vi "Log_Pictures.vi"   [LabVIEW 2017]
uses:
  Anemometry Sub Vis/Controls/Post_Process.ctl
  Anemometry Sub Vis/Globals/Preference_global.vi
  Anemometry Sub Vis/Globals/Extra_Commands_Global.vi
  Anemometry Sub Vis/Globals/Meas_global.vi
  Anemometry Sub Vis/Globals/Trav_pos_global.vi
types:
  T1 = typedef "Post_Process.ctl" = enum16{"Take New Data", "Post Process Raw Data File"}
  T2 = typedef "Camera resolution.ctl" = u8
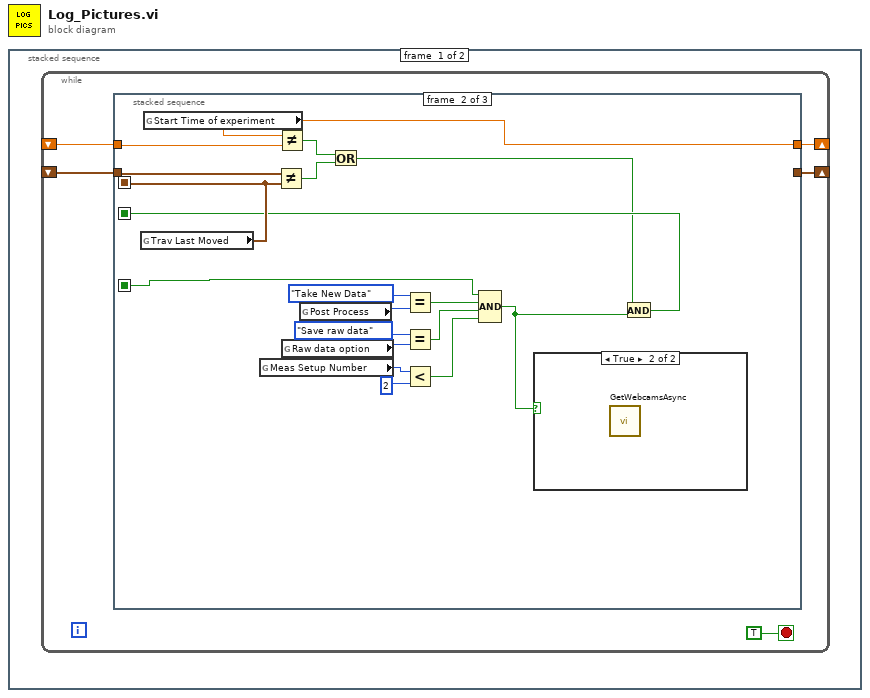
[diagram p0: block diagram]
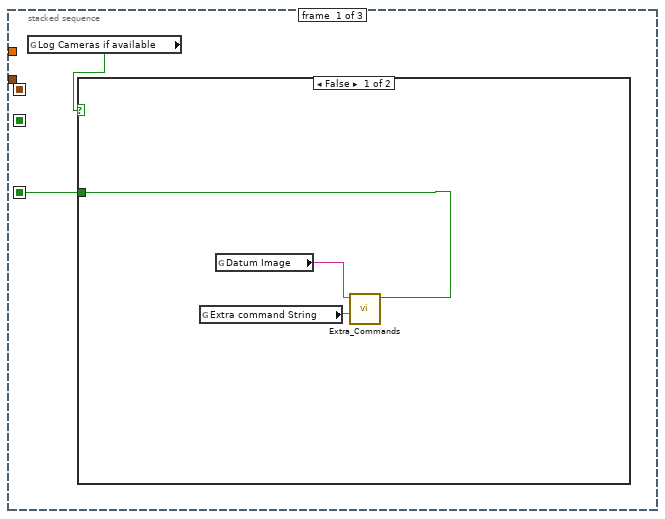
[diagram p2: hidden frame]
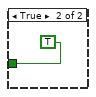
[diagram p3: hidden frame]
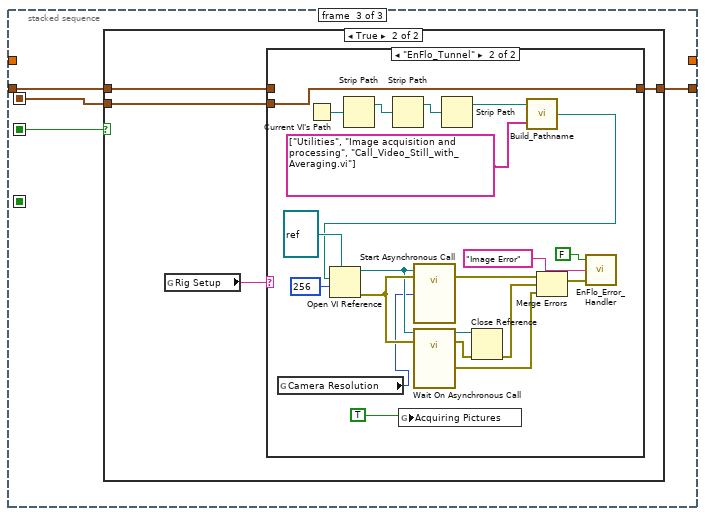
[diagram p5: hidden frame]
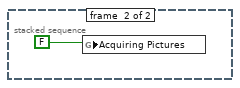
[diagram p8: hidden frame]
diagram:
  n1 = stacked-sequence {
    frame #0 {
      n2 = while {
        shift-right: [w5] -> _
        shift-left: _ -> [w4]
        shift-right: [w2] -> _
        shift-left: _ -> [w3]
        stop <- TRUE stop-if-true
        n3 = stacked-sequence {
          seq-local: [_ w15 _] -> [_ _ w34]
          seq-local: [_ w18 _] -> [_ _ w31]
          seq-local: [w6 _ _] -> [_ w12 _]
          tunnel: [_ _ w33] -> w5
          tunnel: w4 -> [_ w22 w32]
          tunnel: w3 -> [_ w21 _]
          tunnel: [_ w17 _] -> w2
          frame #0 {
            n4 = global read "Preference_global.vi" "Log Cameras if available"() -> (w7:bool)
            n5 = case shown="False" w7 {
              tunnel: [w8 TRUE] -> w6
              frame False {
                n6 = global read "Meas_global.vi" "Extra command String"() -> (w10:string)
                n7 = global read "Extra_Commands_Global.vi" "Datum Image"() -> (w9:string)
                n8 = call "Extra_Commands.vi"("String to Search"=w10, "Command"=w9) -> ("Command Found"=w8:bool)  [unwired: 2 in, 3 out]
              }
              frame True {
              }
            }
          }
          frame #1 {
            n9 = global read "Trav_pos_global.vi" "Trav Last Moved"() -> (w18:timestamp)
            n10 = global read "Meas_global.vi" "Start Time of experiment"() -> (w17:dbl)
            n11 = global read "Trav_pos_global.vi" "Meas Setup Number"() -> (w24:i32)
            n12 = Not Equal?(x=w22, y=w18) -> (x != y?=w19:bool)
            n13 = Not Equal?(x=w17, y=w21) -> (x != y?=w20:bool)
            n14 = global read "Meas_global.vi" "Raw data option"() -> (w27:enum16{"Save raw data", "Raw data not saved"})
            n15 = global read "Meas_global.vi" "Post Process"() -> (w30:T1)
            n16 = Or(x=w20, y=w19) -> (x .or. y?=w14:bool)
            n17 = Equal?(x=Post_Process."Take New Data" ("Post Process"), y=w30) -> (x = y?=w28:bool)
            n18 = Equal?(x=enum16{"Save raw data", "Raw data not saved"}."Save raw data" ("Raw data option"), y=w27) -> (x = y?=w25:bool)
            n19 = Less?(x=w24, y=2) -> (x < y?=w16:bool)
            n20 = Compound Arithmetic op=AND(w12, w28, w25, w16) -> (w13:bool)
            n21 = case shown="True" w13 {
              frame False {
              }
              frame True {
                n22 = call "GetWebcamsAsync.vi"() -> ()  [unwired: 12 in]
              }
            }
            n23 = And(x=w14, y=w13) -> (x .and. y?=w15:bool)
          }
          frame #2 {
            n24 = case shown="True" w34 {
              tunnel: [w35 w38] -> w33
              tunnel: w32 -> [w35 w37]
              tunnel: w31 -> [_ w36]
              frame False {
              }
              frame True {
                n25 = global read "Preference_global.vi" "Rig Setup"() -> (w39:string)
                n26 = case shown="\"EnFlo_Tunnel\"" w39 {
                  tunnel: [w40 w53] -> w38
                  tunnel: w37 -> [w40 _]
                  tunnel: w36 -> [_ w53]
                  frame "False", Default {
                  }
                  frame "EnFlo_Tunnel" {
                    n27 = global read "Meas_global.vi" "Camera Resolution"() -> (w47:T2)
                    n28 = Current VI's Path() -> (path=w61:path)
                    n29 = Strip Path(path=w61) -> (stripped path=w43:path)  [unwired: 1 out]
                    n30 = Strip Path(path=w43) -> (stripped path=w42:path)  [unwired: 1 out]
                    n31 = global write "Meas_global.vi" "Acquiring Pictures"(TRUE) -> ()
                    n32 = Strip Path(path=w42) -> (stripped path=w41:path)  [unwired: 1 out]
                    n33 = call "Build_Pathname.vi"("PathElements"=string[] ["Utilities", "Image acquisition and processing", "Call_Video_Still_with_Averaging.vi"], "PathnameIn"=w41) -> ("AppendedPath"=w46:path)
                    n34 = Open VI Reference(type specifier VI Refnum (for type only)=refnum<vi> refnum, vi path=w46, options=256) -> (vi reference=w48:refnum<vi>, error out=w58:errorcluster)  [unwired: 3 in]
                    n35 = call-by-ref "Start Asynchronous Call"(reference=w48, error in=w58, "Resolution"=w47) -> (error out=w55:errorcluster)  [unwired: 1 in, 2 out]
                    n36 = call-by-ref "Wait On Asynchronous Call"(reference=w48, error in=w58) -> (reference out=w57:refnum<vi>, error out=w56:errorcluster, "Error out"=w52:errorcluster)  [unwired: 2 in]
                    n37 = Close Reference(reference=w57, error in (no error)=w56) -> (error out=w54:errorcluster)
                    n38 = Merge Errors(w55, w54, w52) -> (w50:errorcluster)
                    n39 = call "EnFlo_Error_Handler.vi"("error in (no error)"=w50, "Error Type"="Image Error", "Dialog Box (T)"=FALSE) -> ()  [unwired: 3 out]
                  }
                }
              }
            }
          }
        }
      }
    }
    frame #1 {
      n40 = global write "Meas_global.vi" "Acquiring Pictures"(FALSE) -> ()
    }
  }
